vi "Autonomous Independent.vi"   [LabVIEW 2018]
doc: "This VI is called when autonomous begins, and will automatically be terminated when autonomous ends. You can carry out timed or sensor driven robot movement independently without needing to return to the caller."
uses:
  <vilib>/Rock Robotics/WPI/Solenoid/WPI_SolenoidValue.ctl
  <vilib>/Rock Robotics/Network Tables/NT Read String.vi
  <vilib>/Rock Robotics/Network Tables/NT Read Number.vi
  <vilib>/Rock Robotics/WPI/Utilities/WPI_GetSetVariantRefNum.vi
  Robot Global Data.vi
  <vilib>/Rock Robotics/Network Tables/NT Write Numeric Array.vi
  <vilib>/Rock Robotics/WPI/Solenoid/WPI_SolenoidSetEnum.vi
  <vilib>/Rock Robotics/WPI/RobotDrive/WPI_RobotDriveArcadeDrive_Standard(NoSaturation).vi
panel:
  # "Be sure to right-click and choose Data Operations>>Make Current Value default if you want to save the array values with the VI"
types:
  T1 = typedef "WPI_SolenoidValue.ctl" = enum16{"Off", "On", "Forward", "Reverse"}
  T2 = typedef "WPI_JoystickDevRef.ctl" = cluster{"Device":T3}
  T3 = typedef "WPI_JoystickDeviceEnum.ctl" = enum16{"USB 0", "USB 1", "USB 2", "USB 3", "USB 4", "USB 5"}
  T4 = typedef "WPI_DriverStationPositionInfo.ctl" = enum16{"1", "2", "3"}
  T5 = typedef "WPI_DriverStationAllianceInfo.ctl" = enum16{"Red", "Blue", "Invalid"}
  T6 = typedef "WPI_SolenoidDevRef.ctl" = cluster{"DevStatus":errorcluster, "Pneumatics Control Module":u8, "Forward Solenoid Channel":T7, "Reverse Solenoid Channel":T7}
  T7 = typedef "WPI_SolenoidChannel.ctl" = enum8{"Solenoid 0", "Solenoid 1", "Solenoid 2", "Solenoid 3", "Solenoid 4", "Solenoid 5", "Solenoid 6", "Solenoid 7", "Invalid"}
  T8 = typedef "WPI_RobotDriveDevRef.ctl" = cluster{"DevStatus":errorcluster, "Motors[]":T9[], "Square Inputs":bool, "Max Output":dbl}
  T9 = typedef "WPI_MotorControlDeviceRef.ctl" = cluster{"DeviceStatus":errorcluster, "Type":T10, "PWM":cluster{"PWM Channel":T11, "DeadBand":T12}, "CAN":cluster{"Device Number":u8, "SetOutput VI Ref":variant, "GetOutput VI Ref":variant, "Enable VI Ref":variant, "Disable VI Ref":variant, "Data":variant}, "Invert":bool, "DIO PWM":cluster{"PWM \"Enable\" Channel":T11, "DIOChannel":T13, "PWM Rate":dbl}}
  T10 = typedef "WPI_MotorControlType.ctl" = enum16{"PWM", "CAN", "DIO PWM"}
  T11 = typedef "FPGA_DIOPWMChannel.ctl" = enum8{"PWM 0", "PWM 1", "PWM 2", "PWM 3", "PWM 4", "PWM 5", "PWM 6", "PWM 7", "PWM 8", "PWM 9", "PWM MXP 0", "PWM MXP 1", "PWM MXP 2", "PWM MXP 3", "PWM MXP 4", "PWM MXP 5", "PWM MXP 6", "PWM MXP 7", "PWM MXP 8", "PWM MXP 9", "Invalid"}
  T12 = typedef "WPI_PWMDeadband.ctl" = cluster{"Name":string, "maxPositivePwm":i32, "minPositivePwm":i32, "centerPwm":i32, "maxNegativePwm":i32, "minNegativePwm":i32, "angularRange":u16}
  T13 = typedef "FPGA_DIOChannel.ctl" = enum8{"DIO 0", "DIO 1", "DIO 2", "DIO 3", "DIO 4", "DIO 5", "DIO 6", "DIO 7", "DIO 8", "DIO 9", "DIO MXP 0", "DIO MXP 1", "DIO MXP 2", "DIO MXP 3", "DIO MXP 4", "DIO MXP 5", "DIO MXP 6", "DIO MXP 7", "DIO MXP 8", "DIO MXP 9", "DIO MXP 10", "DIO MXP 11", "DIO MXP 12", "DIO MXP 13", "DIO MXP 14", "DIO MXP 15", "SPI Port CS1", "SPI Port CS2", "SPI Port CS3", "SPI Port MISO", "SPI Port MOSI", "Invalid"}
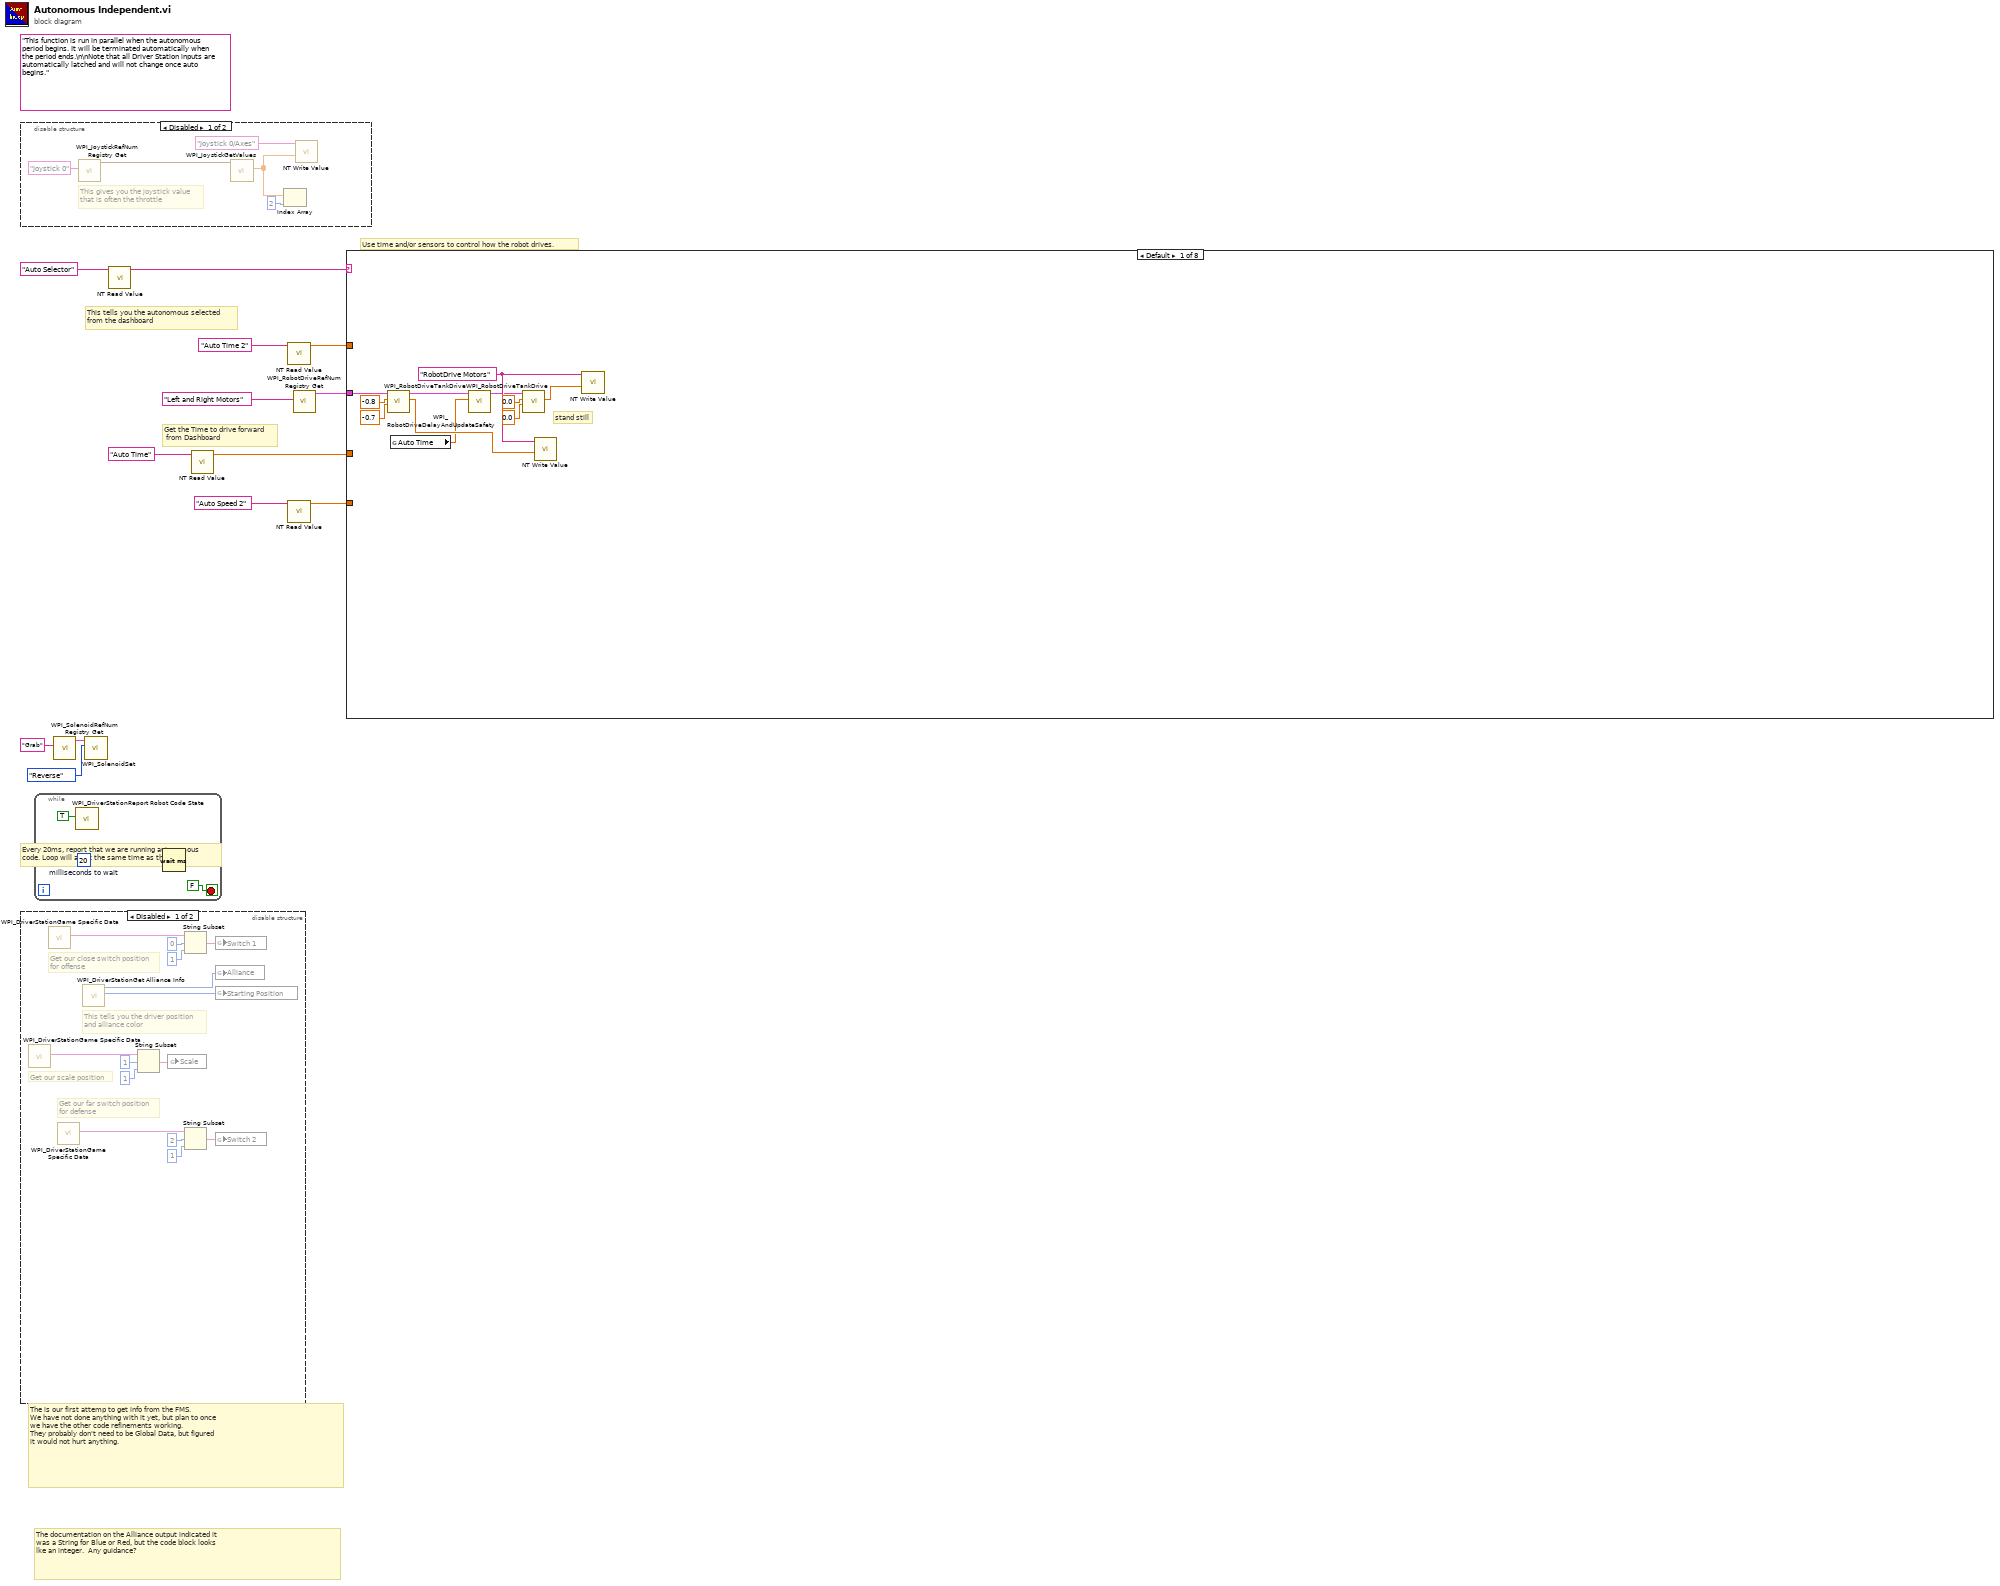
[diagram p0: block diagram]
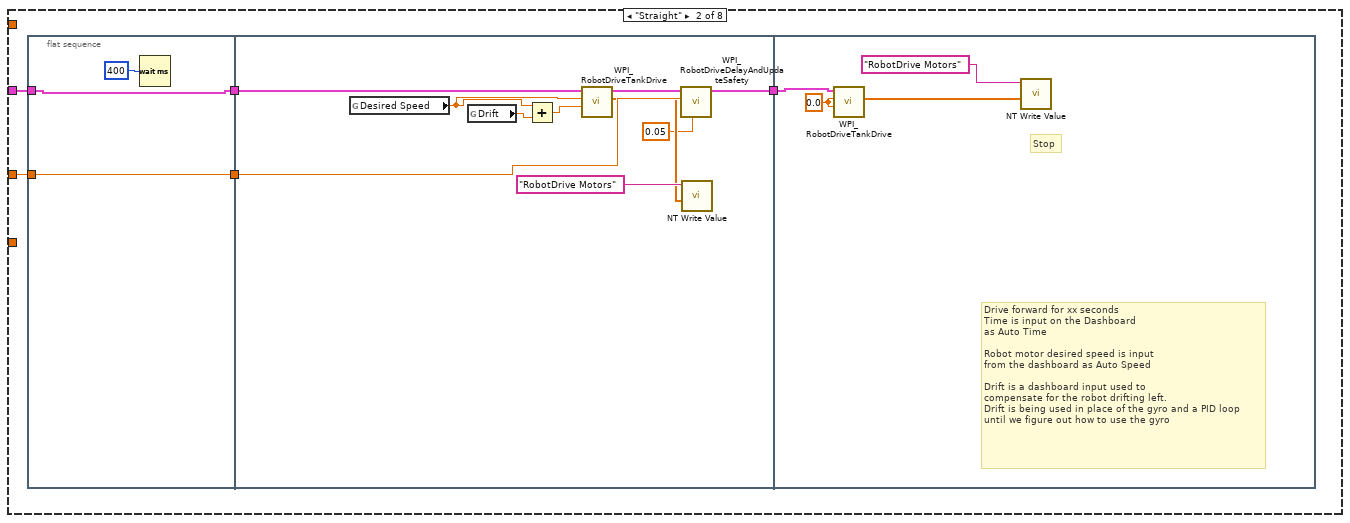
[diagram p4: hidden frame]
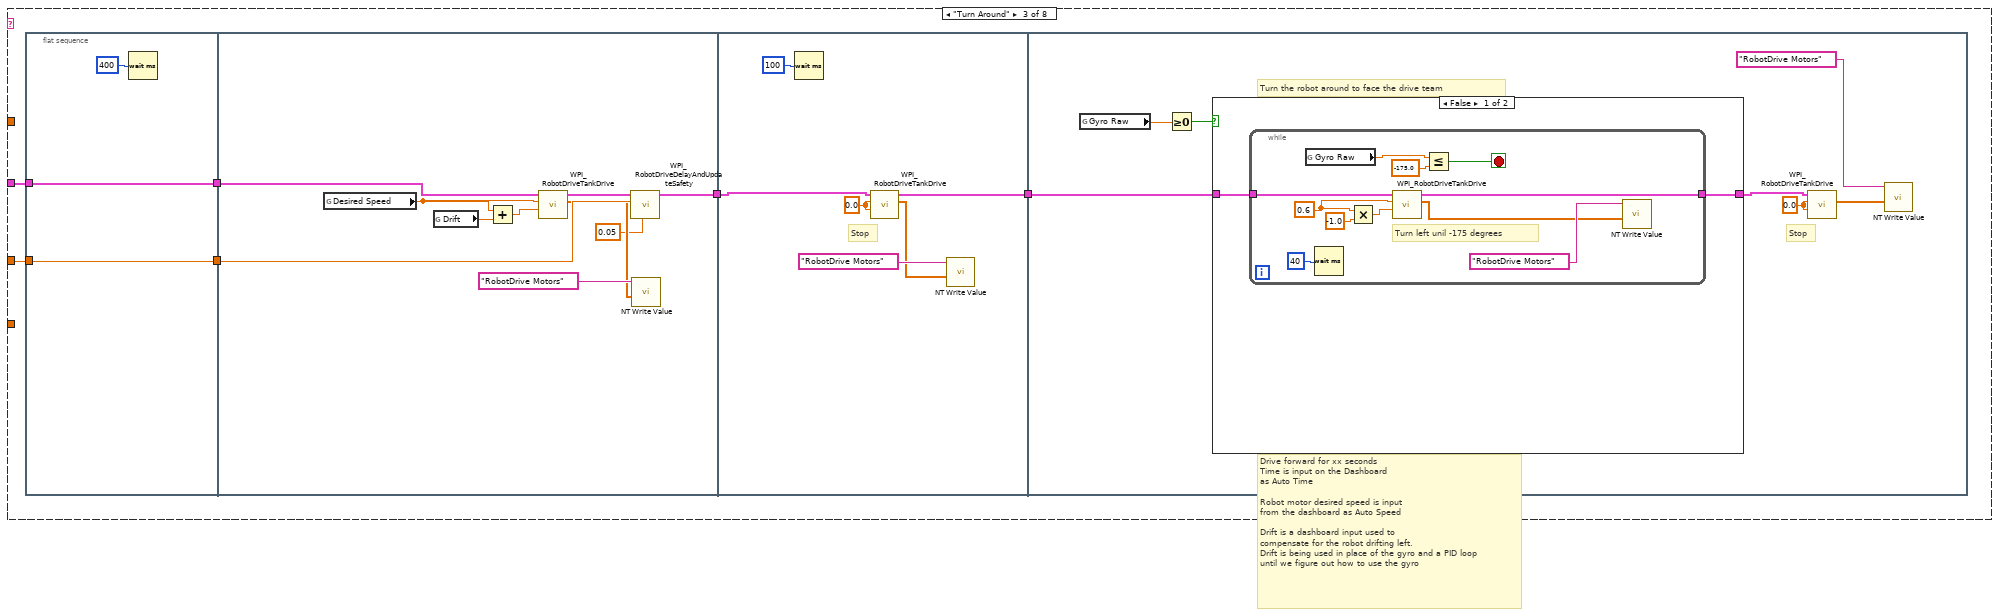
[diagram p5: hidden frame]
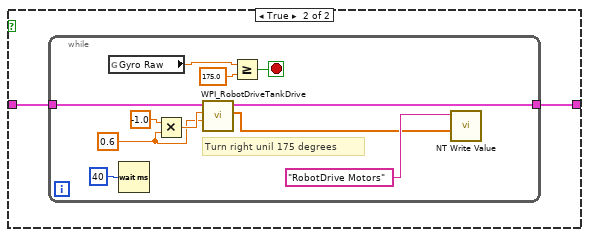
[diagram p6: hidden frame]
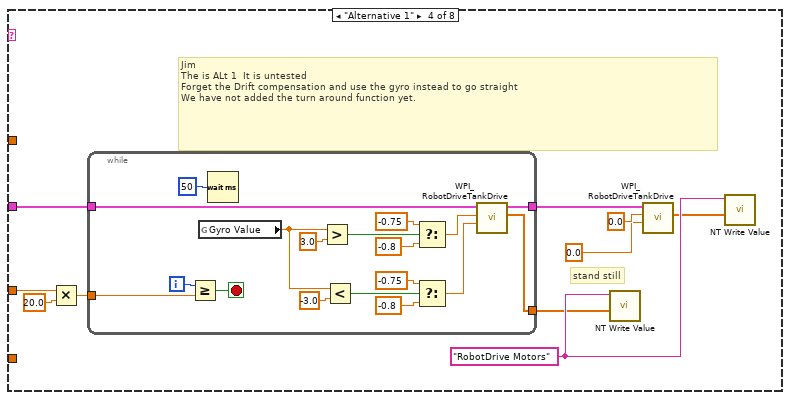
[diagram p7: hidden frame]
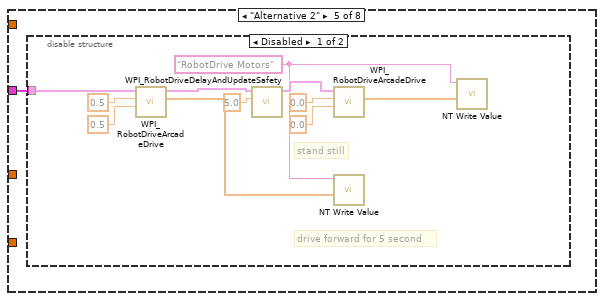
[diagram p8: hidden frame]
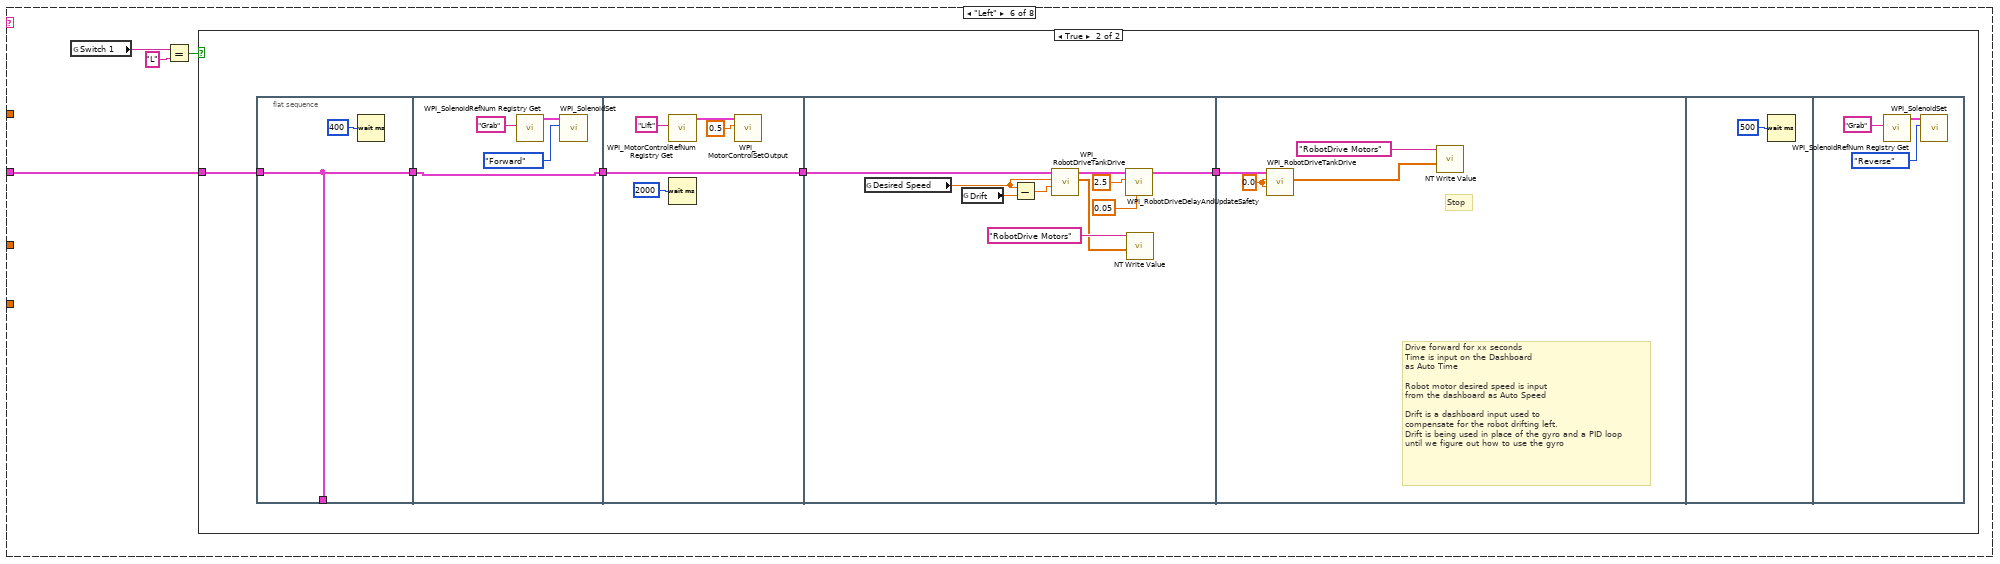
[diagram p10: hidden frame]
diagram:
  (unwired) "This function is run in parallel when the autonomous period begins. It will be terminated automatically when the period ends.\n\nNote that all Driver Station inputs are automatically latched and will not change once auto begins."
  # "The documentation on the Alliance output indicated it\nwas a String for Blue or Red, but the code block looks\nlke an integer.  Any guidance?"
  # "The is our first attemp to get info from the FMS.\nWe have not done anything with it yet, but plan to once\nwe have the other code refinements working.\nThey probably don't need to be Global Data, but figured\nit would not hurt anything."
  # "Get the Time to drive forward\n from Dashboard"
  # "This tells you the autonomous selected\nfrom the dashboard"
  # "Use time and/or sensors to control how the robot drives."
  n1 = disable-structure shown="Disabled" {
    frame Disabled {
      # "This gives you the joystick value\nthat is often the throttle"
      n2 = call <vilib>:"WPI_JoystickRefNum Registry Get.vi"("refnum name"="Joystick 0") -> ("JoystickDevRef"=w17:T2)  [unwired: 1 in, 9 out]
      n3 = call <vilib>:"WPI_JoystickGetValues.vi"("JoystickDevRef"=w17) -> ("Axes"=w15:dbl[])  [unwired: 6 in, 4 out]
      n4 = Index Array(array=w15, index=2) -> ()  [unwired: 1 out]
      n5 = call-poly <vilib>:"NT Write Value.vi"("Numeric Array"=w15, "Name"="Joystick 0/Axes") -> ()  [unwired: 9 in, 1 out]
    }
    frame Enabled {
    }
  }
  n6 = disable-structure shown="Disabled" {
    frame Disabled {
      # "Get our scale position"
      # "Get our far switch position\nfor defense"
      # "Get our close switch position\nfor offense"
      # "This tells you the driver position\nand alliance color"
      n7 = call <vilib>:"WPI_DriverStationGame Specific Data.vi"() -> ("Game Specific Data"=w27:string)  [unwired: 11 in]
      n8 = call <vilib>:"WPI_DriverStationGame Specific Data.vi"() -> ("Game Specific Data"=w32:string)  [unwired: 11 in]
      n9 = call <vilib>:"WPI_DriverStationGame Specific Data.vi"() -> ("Game Specific Data"=w26:string)  [unwired: 11 in]
      n10 = call <vilib>:"WPI_DriverStationGet Alliance Info.vi"() -> ("Position"=w20:T4, "Alliance"=w19:T5)  [unwired: 10 out]
      n11 = String Subset(string=w27, offset (0)=1, length (rest)=1 ("length (rest)")) -> (substring=w22:string)
      n12 = global write "Robot Global Data.vi" "Scale"(w22) -> ()
      n13 = String Subset(string=w32, offset (0)=0, length (rest)=1 ("length (rest)")) -> (substring=w23:string)
      n14 = String Subset(string=w26, offset (0)=2, length (rest)=1 ("length (rest)")) -> (substring=w21:string)
      n15 = global write "Robot Global Data.vi" "Switch 1"(w23) -> ()
      n16 = global write "Robot Global Data.vi" "Alliance"(w19) -> ()
      n17 = global write "Robot Global Data.vi" "Starting Position"(w20) -> ()
      n18 = global write "Robot Global Data.vi" "Switch 2"(w21) -> ()
    }
    frame Enabled {
    }
  }
  n19 = while {
    stop <- FALSE stop-if-true
    w33 = u32 20  # milliseconds to wait
    # "Every 20ms, report that we are running autonomous\ncode. Loop will abort the same time as the VI."
    n20 = call <vilib>:"WPI_DriverStationReport Robot Code State.vi"("Autonomous"=TRUE) -> ()  [unwired: 10 in, 1 out]
    n21 = Wait (ms)(milliseconds to wait=w33) -> ()  [unwired: 1 out]
  }
  n22 = call <vilib>:"WPI_SolenoidRefNum Registry Get.vi"("refnum name"="Grab") -> ("SolenoidDevRef"=w1:T6)  [unwired: 9 in, 1 out]
  n23 = call-poly <vilib>:"WPI_SolenoidSet.vi"("Value"=WPI_SolenoidValue."Reverse", "SolenoidDevRef"=w1) -> ()  [unwired: 8 in, 2 out]
  n24 = call-poly <vilib>:"NT Read Value.vi"("Name"="Auto Selector") -> ("String"=w12:string)  [unwired: 9 in, 1 out]
  n25 = call-poly <vilib>:"NT Read Value.vi"("Name"="Auto Time") -> ("Numeric"=w10:dbl)  [unwired: 9 in, 1 out]
  n26 = call-poly <vilib>:"NT Read Value.vi"("Name"="Auto Time 2") -> ("Numeric"=w4:dbl)  [unwired: 9 in, 1 out]
  n27 = call-poly <vilib>:"NT Read Value.vi"("Name"="Auto Speed 2") -> ("Numeric"=w5:dbl)  [unwired: 9 in, 1 out]
  n28 = call <vilib>:"WPI_RobotDriveRefNum Registry Get.vi"("refnum name"="Left and Right Motors") -> ("RobotDriveDevRef"=w8:T8)  [unwired: 1 in, 9 out]
  n29 = case shown="Default" w12 {
    tunnel: w10 -> [_ w50 w73 w128 _ _ _ _]
    tunnel: w8 -> [w45 w51 w74 w127 w155 w170 _ _]
    tunnel: w5 -> [_ _ _ _ _ _ _ _]
    tunnel: w4 -> [_ _ _ _ _ _ _ _]
    frame Default {
      w46 = "RobotDrive Motors" ("Name")
      # "stand still"
      n30 = call <vilib>:"WPI_RobotDriveTankDrive.vi"("Right axis value"=-0.7 ("X axis value"), "Left axis value"=-0.8, "RobotDriveDevRef"=w45) -> ("Motor Values"=w44:dbl[], "RobotDriveDevRef"=w43:T8)  [unwired: 6 in, 1 out]
      n31 = global read "Robot Global Data.vi" "Auto Time"() -> (w36:dbl)
      n32 = call <vilib>:"WPI_RobotDriveDelayAndUpdateSafety.vi"("Delay (s)"=w36, "RobotDriveDevRef"=w43) -> ("RobotDriveDevRef 2"=w42:T8)  [unwired: 8 in, 1 out]
      n33 = call <vilib>:"WPI_RobotDriveTankDrive.vi"("Right axis value"=0.0 ("X axis value"), "Left axis value"=0.0 ("X axis value"), "RobotDriveDevRef"=w42) -> ("Motor Values"=w39:dbl[])  [unwired: 6 in, 2 out]
      n34 = call-poly <vilib>:"NT Write Value.vi"("Numeric Array"=w44, "Name"=w46) -> ()  [unwired: 9 in, 1 out]
      n35 = call-poly <vilib>:"NT Write Value.vi"("Numeric Array"=w39, "Name"=w46) -> ()  [unwired: 9 in, 1 out]
    }
    frame "Straight" {
      n36 = flat-sequence {
        tunnel: w50 -> [w53]
        tunnel: w51 -> [w54]
        tunnel: [w54] -> w48
        tunnel: [w53] -> w47
        tunnel: [w57] -> w49
        tunnel: w48 -> [w61]
        tunnel: w47 -> [w60]
        tunnel: w49 -> [w65]
        frame #0 {
          n37 = Wait (ms)(milliseconds to wait=u32 400) -> ()  [unwired: 1 out]
        }
        frame #1 {
          n38 = global read "Robot Global Data.vi" "Desired Speed"() -> (w55:dbl)
          n39 = global read "Robot Global Data.vi" "Drift"() -> (w62:dbl)
          n40 = Add(x=w55, y=w62) -> (x+y=w63:dbl)
          n41 = call <vilib>:"WPI_RobotDriveTankDrive.vi"("Right axis value"=w63, "Left axis value"=w55, "RobotDriveDevRef"=w61) -> ("Motor Values"=w58:dbl[], "RobotDriveDevRef"=w64:T8)  [unwired: 6 in, 1 out]
          n42 = call <vilib>:"WPI_RobotDriveDelayAndUpdateSafety.vi"("Feed time (s)"=0.05, "Delay (s)"=w60, "RobotDriveDevRef"=w64) -> ("RobotDriveDevRef 2"=w57:T8)  [unwired: 7 in, 1 out]
          n43 = call-poly <vilib>:"NT Write Value.vi"("Numeric Array"=w58, "Name"="RobotDrive Motors") -> ()  [unwired: 9 in, 1 out]
        }
        frame #2 {
          w68 = 0.0 ("Right axis value")
          # "Drive forward for xx seconds\nTime is input on the Dashboard\nas Auto Time\n\nRobot motor desired speed is input\nfrom the dashboard as Auto Speed\n\nDrift is a dashboard input used to\ncompensate for the robot drifting left.\nDrift is being used in place of the gyro and a PID loop\nuntil we figure out how to use the gyro"
          # "Stop"
          n44 = call <vilib>:"WPI_RobotDriveTankDrive.vi"("Right axis value"=w68, "Left axis value"=w68, "RobotDriveDevRef"=w65) -> ("Motor Values"=w66:dbl[])  [unwired: 6 in, 2 out]
          n45 = call-poly <vilib>:"NT Write Value.vi"("Numeric Array"=w66, "Name"="RobotDrive Motors") -> ()  [unwired: 9 in, 1 out]
        }
      }
    }
    frame "Turn Around" {
      n46 = flat-sequence {
        tunnel: w73 -> [w76]
        tunnel: w74 -> [w77]
        tunnel: [w77] -> w70
        tunnel: [w76] -> w69
        tunnel: [w80] -> w72
        tunnel: w70 -> [w84]
        tunnel: w69 -> [w83]
        tunnel: w72 -> [w91]
        tunnel: [w89] -> w71
        tunnel: w71 -> [w94]
        frame #0 {
          n47 = Wait (ms)(milliseconds to wait=u32 400) -> ()  [unwired: 1 out]
        }
        frame #1 {
          n48 = global read "Robot Global Data.vi" "Desired Speed"() -> (w78:dbl)
          n49 = global read "Robot Global Data.vi" "Drift"() -> (w85:dbl)
          n50 = Add(x=w78, y=w85) -> (x+y=w86:dbl)
          n51 = call <vilib>:"WPI_RobotDriveTankDrive.vi"("Right axis value"=w86, "Left axis value"=w78, "RobotDriveDevRef"=w84) -> ("Motor Values"=w81:dbl[], "RobotDriveDevRef"=w87:T8)  [unwired: 6 in, 1 out]
          n52 = call <vilib>:"WPI_RobotDriveDelayAndUpdateSafety.vi"("Feed time (s)"=0.05, "Delay (s)"=w83, "RobotDriveDevRef"=w87) -> ("RobotDriveDevRef 2"=w80:T8)  [unwired: 7 in, 1 out]
          n53 = call-poly <vilib>:"NT Write Value.vi"("Numeric Array"=w81, "Name"="RobotDrive Motors") -> ()  [unwired: 9 in, 1 out]
        }
        frame #2 {
          w92 = 0.0 ("Right axis value")
          # "Stop"
          n54 = Wait (ms)(milliseconds to wait=u32 100) -> ()  [unwired: 1 out]
          n55 = call <vilib>:"WPI_RobotDriveTankDrive.vi"("Right axis value"=w92, "Left axis value"=w92, "RobotDriveDevRef"=w91) -> ("Motor Values"=w90:dbl[], "RobotDriveDevRef"=w89:T8)  [unwired: 6 in, 1 out]
          n56 = call-poly <vilib>:"NT Write Value.vi"("Numeric Array"=w90, "Name"="RobotDrive Motors") -> ()  [unwired: 9 in, 1 out]
        }
        frame #3 {
          w100 = 0.0 ("Right axis value")
          # "Turn the robot around to face the drive team"
          # "Stop"
          # "Drive forward for xx seconds\nTime is input on the Dashboard\nas Auto Time\n\nRobot motor desired speed is input\nfrom the dashboard as Auto Speed\n\nDrift is a dashboard input used to\ncompensate for the robot drifting left.\nDrift is being used in place of the gyro and a PID loop\nuntil we figure out how to use the gyro"
          n57 = global read "Robot Global Data.vi" "Gyro Raw"() -> (w95:dbl)
          n58 = Greater Or Equal To 0?(x=w95) -> (x >= 0?=w96:bool)
          n59 = case shown="False" w96 {
            tunnel: [w102 w114] -> w99
            tunnel: w94 -> [w101 w115]
            frame False {
              n60 = while {
                tunnel: [w113] -> w102
                tunnel: w101 -> [w107]
                stop <- w112 stop-if-true
                w104 = 0.6 ("Left axis value")
                # "Turn left unil -175 degrees"
                n61 = global read "Robot Global Data.vi" "Gyro Raw"() -> (w110:dbl)
                n62 = Wait (ms)(milliseconds to wait=u32 40) -> ()  [unwired: 1 out]
                n63 = Multiply(x=w104, y=-1.0) -> (x*y=w106:dbl)
                n64 = call <vilib>:"WPI_RobotDriveTankDrive.vi"("Right axis value"=w106, "Left axis value"=w104, "RobotDriveDevRef"=w107) -> ("Motor Values"=w108:dbl[], "RobotDriveDevRef"=w113:T8)  [unwired: 6 in, 1 out]
                n65 = Less Or Equal?(x=w110, y=-175.0) -> (x <= y?=w112:bool)
                n66 = call-poly <vilib>:"NT Write Value.vi"("Numeric Array"=w108, "Name"="RobotDrive Motors") -> ()  [unwired: 9 in, 1 out]
              }
            }
            frame True {
              n67 = while {
                tunnel: [w126] -> w114
                tunnel: w115 -> [w120]
                stop <- w125 stop-if-true
                w117 = 0.6 ("Left axis value")
                # "Turn right unil 175 degrees"
                n68 = global read "Robot Global Data.vi" "Gyro Raw"() -> (w123:dbl)
                n69 = Wait (ms)(milliseconds to wait=u32 40) -> ()  [unwired: 1 out]
                n70 = Multiply(x=-1.0, y=w117) -> (x*y=w119:dbl)
                n71 = call <vilib>:"WPI_RobotDriveTankDrive.vi"("Right axis value"=w117, "Left axis value"=w119, "RobotDriveDevRef"=w120) -> ("Motor Values"=w121:dbl[], "RobotDriveDevRef"=w126:T8)  [unwired: 6 in, 1 out]
                n72 = Greater Or Equal?(x=w123, y=175.0) -> (x >= y?=w125:bool)
                n73 = call-poly <vilib>:"NT Write Value.vi"("Numeric Array"=w121, "Name"="RobotDrive Motors") -> ()  [unwired: 9 in, 1 out]
              }
            }
          }
          n74 = call <vilib>:"WPI_RobotDriveTankDrive.vi"("Right axis value"=w100, "Left axis value"=w100, "RobotDriveDevRef"=w99) -> ("Motor Values"=w97:dbl[])  [unwired: 6 in, 2 out]
          n75 = call-poly <vilib>:"NT Write Value.vi"("Numeric Array"=w97, "Name"="RobotDrive Motors") -> ()  [unwired: 9 in, 1 out]
        }
      }
    }
    frame "Alternative 1" {
      w136 = "RobotDrive Motors" ("Name")
      # "Jim\nThe is ALt 1  It is untested\nForget the Drift compensation and use the gyro instead to go straight\nWe have not added the turn around function yet."
      # "stand still"
      n76 = Multiply(x=w128, y=20.0) -> (x*y=w129:dbl)
      n77 = while {
        tunnel: [w141] -> w131
        tunnel: [w140] -> w132
        tunnel: w129 -> [w139]
        tunnel: w127 -> [w137]
        i -> [w143]
        stop <- w142 stop-if-true
        n78 = Greater Or Equal?(x=w143, y=w139) -> (x >= y?=w142:bool)
        n79 = global read "Robot Global Data.vi" "Gyro Value"() -> (w138:dbl)
        n80 = Wait (ms)(milliseconds to wait=u32 50) -> ()  [unwired: 1 out]
        n81 = Greater?(x=w138, y=3.0) -> (0:w148:bool)
        n82 = Less?(x=w138, y=-3.0) -> (x < y?=w153:bool)
        n83 = Select(t=-0.75, s=w148, f=-0.8) -> (s? t:f=w145:dbl)
        n84 = Select(t=-0.75, s=w153, f=-0.8) -> (s? t:f=w150:dbl)
        n85 = call <vilib>:"WPI_RobotDriveTankDrive.vi"("Right axis value"=w150, "Left axis value"=w145, "RobotDriveDevRef"=w137) -> ("Motor Values"=w140:dbl[], "RobotDriveDevRef"=w141:T8)  [unwired: 6 in, 1 out]
      }
      n86 = call-poly <vilib>:"NT Write Value.vi"("Numeric Array"=w132, "Name"=w136) -> ()  [unwired: 9 in, 1 out]
      n87 = call <vilib>:"WPI_RobotDriveTankDrive.vi"("Right axis value"=0.0 ("X axis value"), "Left axis value"=0.0 ("X axis value"), "RobotDriveDevRef"=w131) -> ("Motor Values"=w133:dbl[])  [unwired: 6 in, 2 out]
      n88 = call-poly <vilib>:"NT Write Value.vi"("Numeric Array"=w133, "Name"=w136) -> ()  [unwired: 9 in, 1 out]
    }
    frame "Alternative 2" {
      n89 = disable-structure shown="Disabled" {
        disable-tunnel: w155 -> [w156 _]
        frame Disabled {
          w157 = "RobotDrive Motors" ("Name")
          # "stand still"
          # "drive forward for 5 second"
          n90 = call-poly <vilib>:"WPI_RobotDriveArcadeDrive.vi"("Y axis value"=0.5 ("X axis value"), "X axis value"=0.5, "RobotDriveDevRef"=w156) -> ("Motor Values"=w160:dbl[], "RobotDriveDevRef"=w166:T8)  [unwired: 1 in, 6 out]
          n91 = call <vilib>:"WPI_RobotDriveDelayAndUpdateSafety.vi"("Delay (s)"=5.0 ("X axis value"), "RobotDriveDevRef"=w166) -> ("RobotDriveDevRef 2"=w159:T8)  [unwired: 8 in, 1 out]
          n92 = call-poly <vilib>:"WPI_RobotDriveArcadeDrive.vi"("Y axis value"=0.0 ("X axis value"), "X axis value"=0.0, "RobotDriveDevRef"=w159) -> ("Motor Values"=w161:dbl[])  [unwired: 1 in, 7 out]
          n93 = call-poly <vilib>:"NT Write Value.vi"("Numeric Array"=w160, "Name"=w157) -> ()  [unwired: 9 in, 1 out]
          n94 = call-poly <vilib>:"NT Write Value.vi"("Numeric Array"=w161, "Name"=w157) -> ()  [unwired: 9 in, 1 out]
        }
        frame Enabled {
        }
      }
    }
    frame "Left" {
      n95 = global read "Robot Global Data.vi" "Switch 1"() -> (w168:string)
      n96 = Equal?(x=w168, y="L") -> (x = y?=w169:bool)
      n97 = case shown="True" w169 {
        tunnel: w170 -> [_ w171]
        frame False {
        }
        frame True {
          n98 = flat-sequence {
            tunnel: [w176] -> _
            tunnel: [w176] -> w175
            tunnel: w171 -> [w176]
            tunnel: w175 -> [w181]
            tunnel: [w181] -> w174
            tunnel: w174 -> [w186]
            tunnel: [w186] -> w173
            tunnel: [w190] -> w172
            tunnel: w173 -> [w193]
            tunnel: w172 -> [w197]
            frame #0 {
              n99 = Wait (ms)(milliseconds to wait=u32 400) -> ()  [unwired: 1 out]
            }
            frame #1 {
              n100 = call <vilib>:"WPI_SolenoidRefNum Registry Get.vi"("refnum name"="Grab") -> ("SolenoidDevRef"=w179:T6)  [unwired: 9 in, 1 out]
              n101 = call-poly <vilib>:"WPI_SolenoidSet.vi"("Value"=WPI_SolenoidValue."Forward", "SolenoidDevRef"=w179) -> ()  [unwired: 8 in, 2 out]
            }
            frame #2 {
              n102 = call <vilib>:"WPI_MotorControlRefNum Registry Get.vi"("refnum name"="Lift") -> ("MotorControlDevRef"=w184:T9)  [unwired: 9 in, 1 out]
              n103 = Wait (ms)(milliseconds to wait=u32 2000) -> ()  [unwired: 1 out]
              n104 = call <vilib>:"WPI_MotorControlSetOutput.vi"("Output"=0.5, "MotorControlDevRef"=w184) -> ()  [unwired: 7 in, 3 out]
            }
            frame #3 {
              n105 = global read "Robot Global Data.vi" "Desired Speed"() -> (w188:dbl)
              n106 = global read "Robot Global Data.vi" "Drift"() -> (w194:dbl)
              n107 = Subtract(x=w188, y=w194) -> (x-y=w195:dbl)
              n108 = call <vilib>:"WPI_RobotDriveTankDrive.vi"("Right axis value"=w195, "Left axis value"=w188, "RobotDriveDevRef"=w193) -> ("Motor Values"=w191:dbl[], "RobotDriveDevRef"=w196:T8)  [unwired: 6 in, 1 out]
              n109 = call <vilib>:"WPI_RobotDriveDelayAndUpdateSafety.vi"("Feed time (s)"=0.05, "Delay (s)"=2.5, "RobotDriveDevRef"=w196) -> ("RobotDriveDevRef 2"=w190:T8)  [unwired: 7 in, 1 out]
              n110 = call-poly <vilib>:"NT Write Value.vi"("Numeric Array"=w191, "Name"="RobotDrive Motors") -> ()  [unwired: 9 in, 1 out]
            }
            frame #4 {
              w200 = 0.0 ("Right axis value")
              # "Drive forward for xx seconds\nTime is input on the Dashboard\nas Auto Time\n\nRobot motor desired speed is input\nfrom the dashboard as Auto Speed\n\nDrift is a dashboard input used to\ncompensate for the robot drifting left.\nDrift is being used in place of the gyro and a PID loop\nuntil we figure out how to use the gyro"
              # "Stop"
              n111 = call <vilib>:"WPI_RobotDriveTankDrive.vi"("Right axis value"=w200, "Left axis value"=w200, "RobotDriveDevRef"=w197) -> ("Motor Values"=w198:dbl[])  [unwired: 6 in, 2 out]
              n112 = call-poly <vilib>:"NT Write Value.vi"("Numeric Array"=w198, "Name"="RobotDrive Motors") -> ()  [unwired: 9 in, 1 out]
            }
            frame #5 {
              n113 = Wait (ms)(milliseconds to wait=u32 500) -> ()  [unwired: 1 out]
            }
            frame #6 {
              n114 = call <vilib>:"WPI_SolenoidRefNum Registry Get.vi"("refnum name"="Grab") -> ("SolenoidDevRef"=w203:T6)  [unwired: 9 in, 1 out]
              n115 = call-poly <vilib>:"WPI_SolenoidSet.vi"("Value"=WPI_SolenoidValue."Reverse", "SolenoidDevRef"=w203) -> ()  [unwired: 8 in, 2 out]
            }
          }
        }
      }
    }
    frame "Middle" {
    }
    frame "Right" {
    }
  }
